vi "svx_Colormap Draw Indication Lines.vi"(0 "color map ref in":refnum<vi>, 1 "speed profile":cluster{"time [s]":dbl[], "speed [rpm]":dbl[]} {"speed [rpm]" format="%.2f"; "time [s]" format="%.2f"}, 2 "new picture 2":picture, 3 "plot type":T3(ring), 4 "Frequency type":dbl[](array[numeric])=[10.0], 5 "Order type":dbl[](array[numeric])=[10.0], 6 "Display Order":bool=TRUE, 7 "orderline setting":T2={"Line"={"Width"=1, "Style"=enum."Solid"}, "color"=0}, 8 "Display Frequency":bool=TRUE, 9 "ordertext setting":T1, 10 "Ordertext":bool=TRUE, 11 "frequencyline setting":T2={"Line"={"Width"=1, "Style"=enum."Solid"}, "color"=0}, 12 "Frequencytext":bool=TRUE, 13 "frequencytext setting":T1) -> (14 "color map ref out":refnum<vi>, 17 "Plot Images:Front":picture)   [LabVIEW 2017, in "SVX Colormap.xctl"]
uses:
  <vilib>/addons/_XControls/Colormap/SVX Colormap.xctl
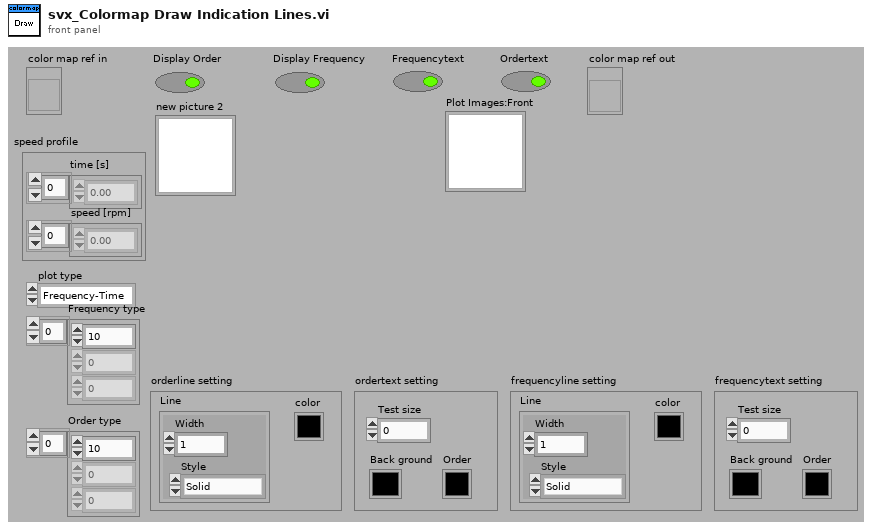
[diagram p1: front panel]
types:
  T1 = cluster{"Test size":i16, "Order":u32, "Back ground":u32}
  T2 = cluster{"Line":cluster{"Width":u16, "Style":enum32{"Solid", "Dash", "Dot", "DashDot", "DashDotDot"}}, "color":u32}
  T3 = enum16{"Frequency-Time", "Time-Frequency", "Order-Time", "Time-Order", "Frequency-RPM", "RPM-Frequency", "Order-RPM", "RPM-Order"}
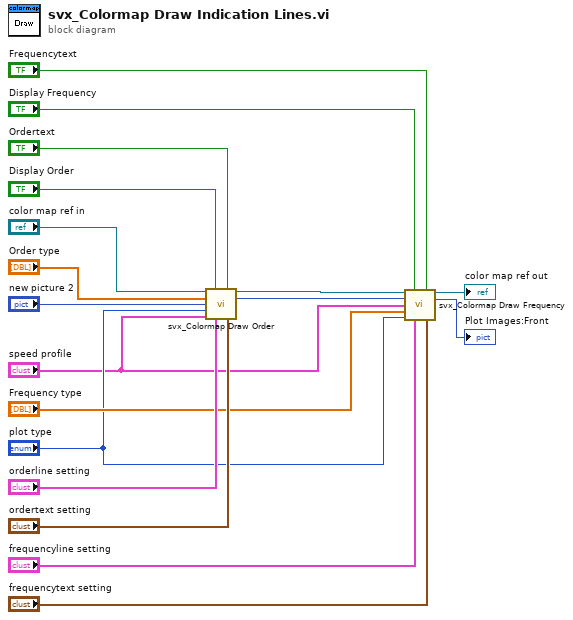
[diagram p0: block diagram]
diagram:
  n1 = call <vilib>:"svx_Colormap Draw Order.vi"("color map ref in"="color map ref in", "Display Order"="Display Order", "Ordertext"="Ordertext", "Order type"="Order type", "new picture 2"="new picture 2", "plot type"="plot type", "speed profile"="speed profile", "Line Configure"="orderline setting", "Text Configure"="ordertext setting") -> ("color map ref out"=w14:refnum<vi>, "new picture"=w13:picture)  [unwired: 5 in]
  n2 = call <vilib>:"svx_Colormap Draw Frequency.vi"("color map ref in"=w14, "Display Frequency"="Display Frequency", "frequencytext"="Frequencytext", "picture in"=w13, "speed profile"="speed profile", "Frequency Type"="Frequency type", "plot type"="plot type", "Line Configure"="frequencyline setting", "Text Configure"="frequencytext setting") -> ("color map ref out"=→"color map ref out":refnum<vi>, "picture out"=→"Plot Images:Front":picture)  [unwired: 5 in]
